vi "Make Waveform.vi"(6 "Number of samples per s":dbl, 7 "Duty cycle (%)":dbl, 9 "405 LED Power":dbl, 10 "470 LED power":dbl, 11 "Frequency":dbl) -> (3 "Array":waveform(dbl)[](array[waveform]))   [LabVIEW 2018]
uses:
  <vilib>/measure/NI_MABase.lvlib
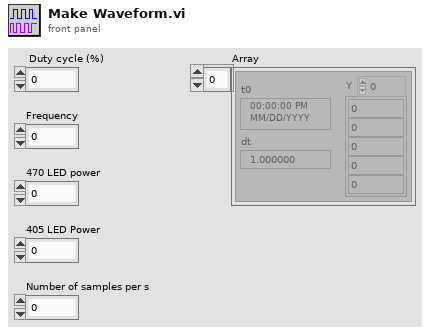
[diagram p1: front panel]
types:
  T1 = enum16{"Sine Wave", "Triangle Wave", "Square Wave", "Sawtooth Wave"}
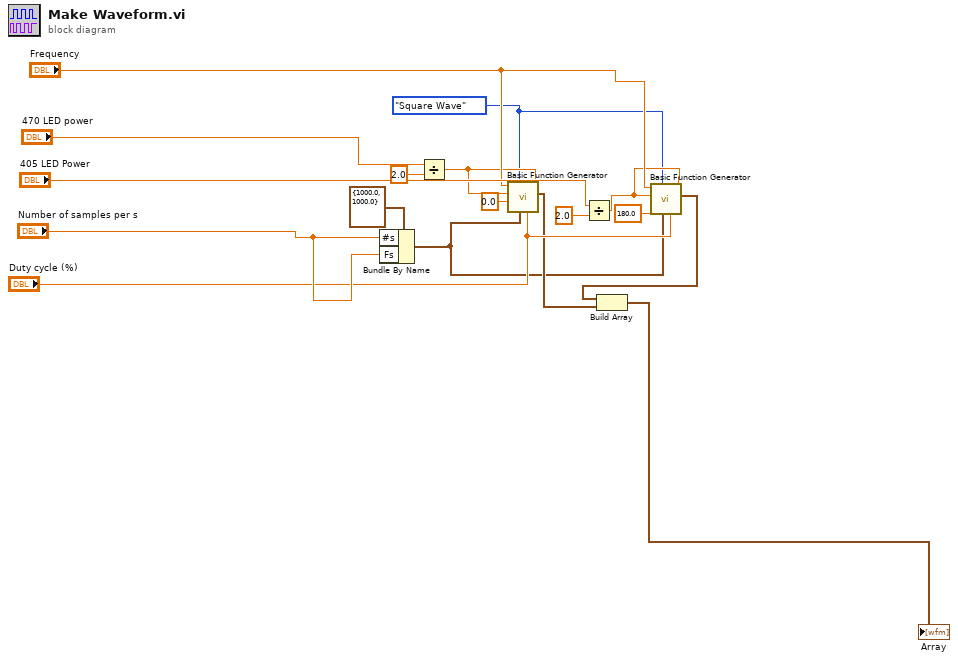
[diagram p0: block diagram]
diagram:
  w2 = T1."Square Wave" ("signal type")
  n1 = Bundle By Name(cluster=cluster{"Fs":dbl, "#s":dbl} {"Fs"=1000.0, "#s"=1000.0} ("sampling info"), "#s"="Number of samples per s", "Fs"="Number of samples per s") -> (w3:cluster{"Fs":dbl, "#s":dbl})
  n2 = Divide(x="470 LED power", y=2.0) -> (x/y=w9:dbl)
  n3 = call <vilib>:"Basic Function Generator.vi"("offset"=w9, "square wave duty cycle (%)"="Duty cycle (%)", "sampling info"=w3, "signal type"=w2, "phase"=0.0, "amplitude"=w9, "frequency"="Frequency") -> ("signal out"=w4:waveform(dbl))  [unwired: 2 in, 2 out]
  n4 = Divide(x="405 LED Power", y=2.0) -> (x/y=w11:dbl)
  n5 = call <vilib>:"Basic Function Generator.vi"("offset"=w11, "square wave duty cycle (%)"="Duty cycle (%)", "sampling info"=w3, "signal type"=w2, "phase"=180.0, "amplitude"=w11, "frequency"="Frequency") -> ("signal out"=w5:waveform(dbl))  [unwired: 2 in, 2 out]
  n6 = Build Array(w5, w4) -> (→"Array":waveform(dbl)[])
